vi "Logger.Variant.DebugAddDmcConfig.vi"() -> ()   [LabVIEW 2016]
uses:
  Logger.Variant.Sets.ctl
  Station/Station.Changeover.State.vi
  Station/Station.Plate.Properties.ctl
  Sequence/Sequence.Code.SerialFormat.ctl
  Drivers/V7310/LowLevel/V7310.Job.Sets.ctl
panel:
  in  "Folder":path=path "C:/Users/szupienko/Desktop"
  out "size(s) 2":i32
  out "size(s)":i32[](array[numeric])
  out "header":string[](array[string])
  out "subarray":string[](array[string])
  in  "VariantSets":T1={"State"=enum."Init", "ImgPath"=path "", "WabcoPlate"="", "WabcoProduct"="", "ClientProduct"="", "ClientPlate"="", "TotalQuantity"=0, "OrderQuantity"=0, "Serial"=0, "Wabco"={"LaserJob"="", "AdditionalTxt"="037", "FactoryCode"="", "RevID"=0, "ForkID"=0, "FailuresLimit"=0, "GlobalCnt"=0, "Bank"=0, "SerialFormat"=enum."6 dig", "CoordA"={"X"=0.0, "Y"=0.0, "Angle"=0.0}, "CoordB"={"X"=0.0, "Y"=0.0, "Angle"=0.0}, "DMCconfig"=0}, "Client"={"LaserJob"="", "AdditionalTxt"="", "FactoryCode"="037", "RevID"=0, "ForkID"=0, "FailuresLimit"=0, "GlobalCnt"=0, "Bank"=0, "SerialFormat"=enum."6 dig", "CoordA"={"X"=0.0, "Y"=0.0, "Angle"=0.0}, "CoordB"={"X"=0.0, "Y"=0.0, "Angle"=0.0}, "DMCconfig"=0}}
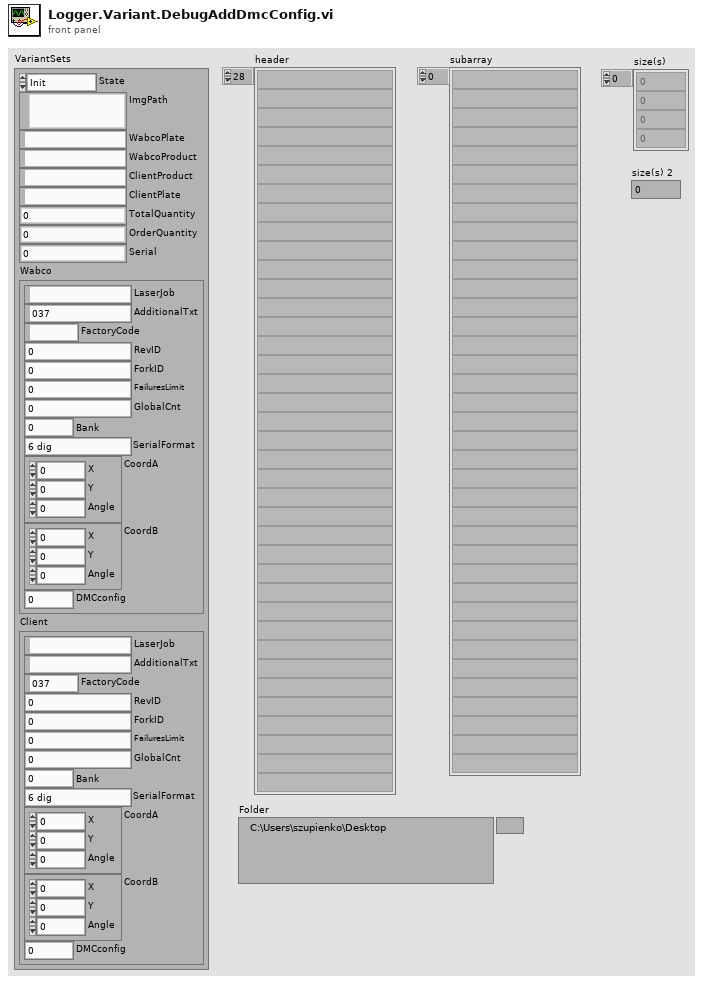
[diagram p1: front panel]
types:
  T1 = typedef "Logger.Variant.Sets.ctl" = cluster{"State":T2, "ImgPath":path, "WabcoPlate":string, "WabcoProduct":string, "ClientProduct":string, "ClientPlate":string, "TotalQuantity":u16, "OrderQuantity":u16, "Serial":i32, "Wabco":T3, "Client":T3}
  T2 = typedef "Station.Changeover.State.vi" = enum16{"Init", "Scaning", "NOK", "Wait for ack", "Ready"}
  T3 = typedef "Station.Plate.Properties.ctl" = cluster{"LaserJob":string, "AdditionalTxt":string, "FactoryCode":string, "RevID":u8, "ForkID":u8, "FailuresLimit":u16, "GlobalCnt":i32, "Bank":u8, "SerialFormat":T4, "CoordA":T5, "CoordB":T5, "DMCconfig":i32}
  T4 = typedef "Sequence.Code.SerialFormat.ctl" = enum8{"", "6 dig", "7 dig"}
  T5 = typedef "V7310.Job.Sets.ctl" = cluster{"X":dbl, "Y":dbl, "Angle":dbl}
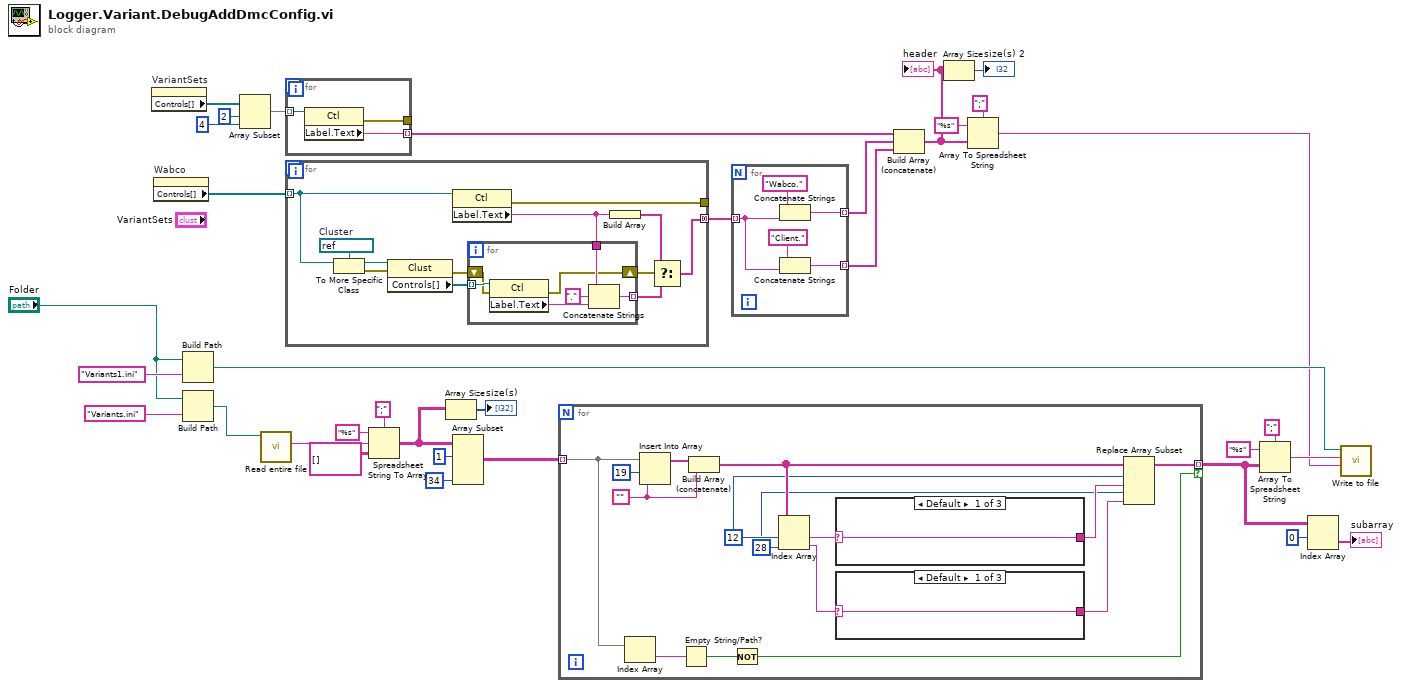
[diagram p0: block diagram]
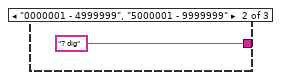
[diagram p2: hidden frame]
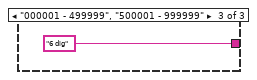
[diagram p3: hidden frame]
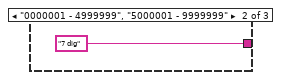
[diagram p4: hidden frame]
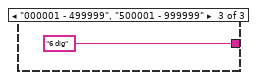
[diagram p5: hidden frame]
diagram:
  n1 = property on="VariantSets" class="Clust (strict)"() -> ("Controls[]"=w17:refnum<vi>[])  [unwired: 2 in, 2 out]
  n2 = property on="Wabco" class="Clust (strict)"() -> ("Controls[]"=w14:refnum<vi>[])  [unwired: 2 in, 2 out]
  n3 = Build Path(base path="Folder", name or relative path="Variants1.ini" ("format string")) -> (appended path=w24:path)
  n4 = Build Path(base path="Folder", name or relative path="Variants.ini" ("format string")) -> (appended path=w33:path)
  n5 = Array Subset(array=w17, index=2, length=4) -> (w16:refnum<vi>[])
  n6 = call "Read entire file.vi"("file"=w33) -> ("contents"=w29:string)  [unwired: 5 in, 1 out]
  n7 = for {
    tunnel: w16 -> [w37] mode=indexing
    tunnel: [w36] -> w20 mode=indexing
    tunnel: [w35] -> _
    n8 = property class="Ctl"(reference=w37) -> (error out=w35:errorcluster, "Label.Text"=w36:string)  [unwired: 1 in, 1 out]
  }
  n9 = for {
    tunnel: w14 -> [w45] mode=indexing
    tunnel: [w38] -> w13 mode=concatenating
    tunnel: [w49] -> _
    w47 = refnum<vi> refnum  # Cluster
    n10 = To More Specific Class(target class=w47, reference=w45) -> (specific class reference=w46:refnum<vi>, error out=w48:errorcluster)  [unwired: 1 in]
    n11 = property class="Clust"(reference=w46, error in=w48) -> (error out=w43:errorcluster, "Controls[]"=w44:refnum<vi>[])  [unwired: 1 out]
    n12 = property class="Ctl"(reference=w45) -> (error out=w49:errorcluster, "Label.Text"=w42:string)  [unwired: 1 in, 1 out]
    n13 = for {
      tunnel: w44 -> [w56] mode=indexing
      tunnel: [w53] -> w39 mode=indexing
      tunnel: w42 -> [w52]
      shift-right: [w50] -> w41
      shift-left: w43 -> [w55]
      n14 = property class="Ctl"(reference=w56, error in=w55) -> (error out=w50:errorcluster, "Label.Text"=w54:string)  [unwired: 1 out]
      n15 = Concatenate Strings(w52, "." ("string"), w54) -> (w53:string)
    }
    n16 = Build Array(w42) -> (w40:string[])
    n17 = Select(t=w40, s=w41, f=w39) -> (s? t:f=w38:string[])
  }
  n18 = Spreadsheet String To Array(delimiter (Tab)=";", format string="%s", spreadsheet string=w29, array type (2D Dbl)=string[][] []) -> (array=w3:string[][])
  n19 = Array Size(array=w3) -> (size(s)=→"size(s)":i32[])
  n20 = Array Subset(array=w3, index (row)=1 ("index"), length (col)=34 ("length")) -> (w2:string[][])  [unwired: 2 in]
  n21 = for {
    tunnel: w2 -> [w64] mode=indexing
    tunnel: [w66] -> w10 mode=indexing if=w61
    w59 = 28 ("index")
    w65 = 12 ("index")
    w69 = ""
    n22 = Index Array(array=w64) -> (element=w63:string)  [unwired: 1 in]
    n23 = Insert Into Array(array=w64, index=19, new element=w69) -> (w70:string[])
    n24 = Empty String/Path?(string/path=w63) -> (empty?=w62:bool)
    n25 = Build Array (concatenate)(w70, w69) -> (w68:string[])
    n26 = Not(x=w62) -> (.not. x?=w61:bool)
    n27 = Index Array(array=w68, index #1=w65, index #2=w59) -> (element #1=w67:string, element #2=w58:string)
    n28 = case shown="Default" w67 {
      selector: w67 -> [w75 _ _]
      tunnel: [w75 "7 dig" "6 dig"] -> w60
      frame Default {
      }
      frame "0000001 - 4999999", "5000001 - 9999999" {
      }
      frame "000001 - 499999", "500001 - 999999" {
      }
    }
    n29 = case shown="Default" w58 {
      selector: w58 -> [w72 _ _]
      tunnel: [w72 "7 dig" "6 dig"] -> w57
      frame Default {
      }
      frame "0000001 - 4999999", "5000001 - 9999999" {
      }
      frame "000001 - 499999", "500001 - 999999" {
      }
    }
    n30 = Replace Array Subset(array=w68, new element #1=w60, index #1=w65, new element #2=w57, index #2=w59) -> (w66:string[])
  }
  n31 = for {
    tunnel: w13 -> [w79] mode=indexing
    tunnel: [w81] -> w12 mode=indexing
    tunnel: [w78] -> w11 mode=indexing
    n32 = Concatenate Strings("Wabco." ("string"), w79) -> (w81:string)
    n33 = Concatenate Strings("Client." ("string"), w79) -> (w78:string)
  }
  n34 = Build Array (concatenate)(w20, w12, w11) -> (w5:string[])
  "header" <- w5
  n35 = Array Size(array=w5) -> (size(s)=→"size(s) 2":i32)
  n36 = Array To Spreadsheet String(delimiter (Tab)=";", array=w5, 3:"%s" ("format string")) -> (spreadsheet string=w15:string)
  n37 = Array To Spreadsheet String(delimiter (Tab)=";", array=w10, 3:"%s" ("format string")) -> (spreadsheet string=w26:string)
  n38 = Index Array(array=w10, index (row)=0) -> (element=→"subarray":string[])  [unwired: 1 in]
  n39 = call "Write to file.vi"("header"=w15, "addition"=w26, "file"=w24) -> ()  [unwired: 8 in, 1 out]
